vi "Test VI Reentrancy.vi"(8 "error in (no error)":errorcluster, 9 "Execution:Reentrancy Type":T1(ring), 10 "VI Refnum":refnum<vi>, 11 "TestCase in":refnum<class "TestCase.lvclass">) -> (0 "error out":errorcluster, 3 "TestCase out":refnum<class "TestCase.lvclass">)   [LabVIEW 2013]
doc: "Test for VI is reentrant and has the reentrancy type specified."
uses:
  <vilib>/addons/_JKI Toolkits/VI Tester/TestCase.llb/TestCase.lvclass
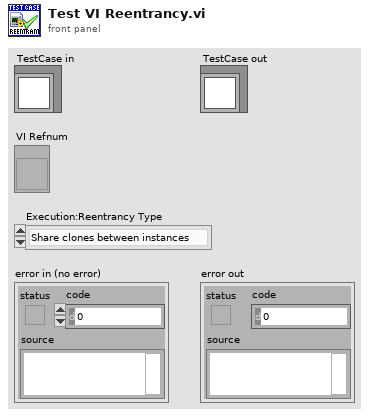
[diagram p1: front panel]
types:
  T1 = enum16{"Share clones between instances", "Preallocate clone for each instance"}
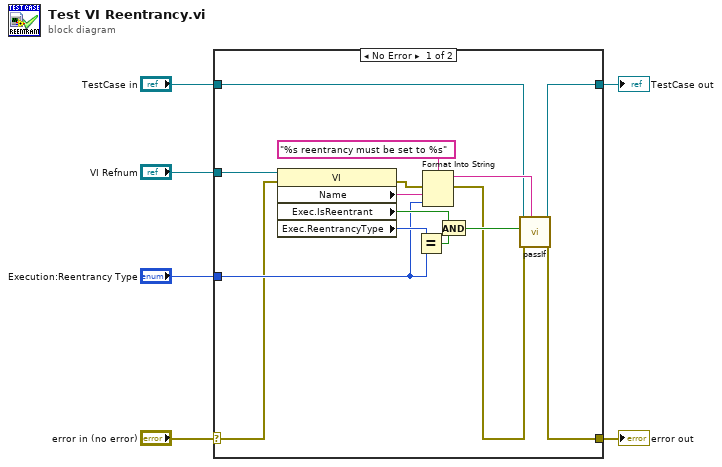
[diagram p0: block diagram]
diagram:
  n1 = case shown="No Error" "error in (no error)" {
    selector: "error in (no error)" -> [w7 w22]
    tunnel: "Execution:Reentrancy Type" -> [w15 _]
    tunnel: [w13 w22] -> w5
    tunnel: "TestCase in" -> [w12 w23]
    tunnel: [w11 w23] -> w3
    tunnel: "VI Refnum" -> [w10 _]
    frame No Error {
      n2 = property class="VI"(reference=w10, error in=w7) -> (error out=w9:errorcluster, "Name"=w17:string, "Exec.IsReentrant"=w20:bool, "Exec.ReentrancyType"=w19:T1)  [unwired: 1 out]
      n3 = Equal?(x=w19, y=w15) -> (x = y?=w21:bool)
      n4 = Format Into String(format string="%s reentrancy must be set to %s" ("custom report message (\"\")"), error in=w9, w17, w15) -> (resulting string=w14:string, error out=w8:errorcluster)  [unwired: 1 in]
      n5 = And(x=w20, y=w21) -> (x .and. y?=w16:bool)
      n6 = call-dynamic "passIf.vi"("custom report message (\"\")"=w14, "error in (no error)"=w8, "pass"=w16, "TestCase in"=w12) -> ("error out"=w13:errorcluster, "TestCase out"=w11:refnum<class "TestCase.lvclass">)  [unwired: 6 in]
    }
    frame Error {
    }
  }
  "error out" <- w5
  "TestCase out" <- w3
